vi "image_acquisitionBYModules.vi"() -> ()   [LabVIEW 2011]
uses:
  state.ctl
panel:
  out "Start acquisition 2":bool
  out "Output \nparameters 2":T2={"Frame rate (ms)"=2000, "Worm strain"="N2", "Time t"=0, "State"=enum."Image acquisition", "Time elapsed"=0.0, "Max_num_runs"=100000, "#TTL"=0, "SD start reference"=100000, "ImSub Value"=0, "Time of last TTL"=0, "Number of Columns"=2, "Number of Rows"=2, "# AdjacentTTL"=0, "Start sleep detection"="", "Sleep Detection"=FALSE, "# Sleep detections"=0, "Time of first sleep detection"=0, "Time max # adjacent TTL"=0, "Image t-1"=[], "Image t"=[]} {"Number of Rows" items=["1"=1, "2"=2, "3"=3, "4"=4]; "Number of Columns" items=["1"=1, "2"=2, "3"=3, "4"=4]}
  in  "Input\nparameters":T3={"Frame rate (ms)"=2000, "Worm Strain"="N2", "Time t"=0, "State"=enum."Image acquisition", "Acquisition time"=0.0, "Maximum # of images"=100000, "#TTL"=0, "time of third ttl "=100000, "ImSub Value"=0, "Time of last TTL"=0, "# Rows"=2, "# Columns"=2, "number of adjacentTTL"=0, "Sleep Deprivation status"="", "Sleep Detection"=FALSE, "Time of first sleep detection"=0, "# Sleep detections"=0, "Time max # adjacent TTL"=-10000, "Image t-1"=[], "Image t"=[]} {"# Columns" items=["1"=1, "2"=2, "3"=3, "4"=4]; "# Rows" items=["1"=1, "2"=2, "3"=3, "4"=4]}
  in  "Frame\nrate (ms)":u32=2000
  out "Intensity Graph 3":u16[][](graph)
  in  "Display\nImage 2":bool
  # "General settings"
  # "Select number of animals"
  # "Row"
  # "Column"
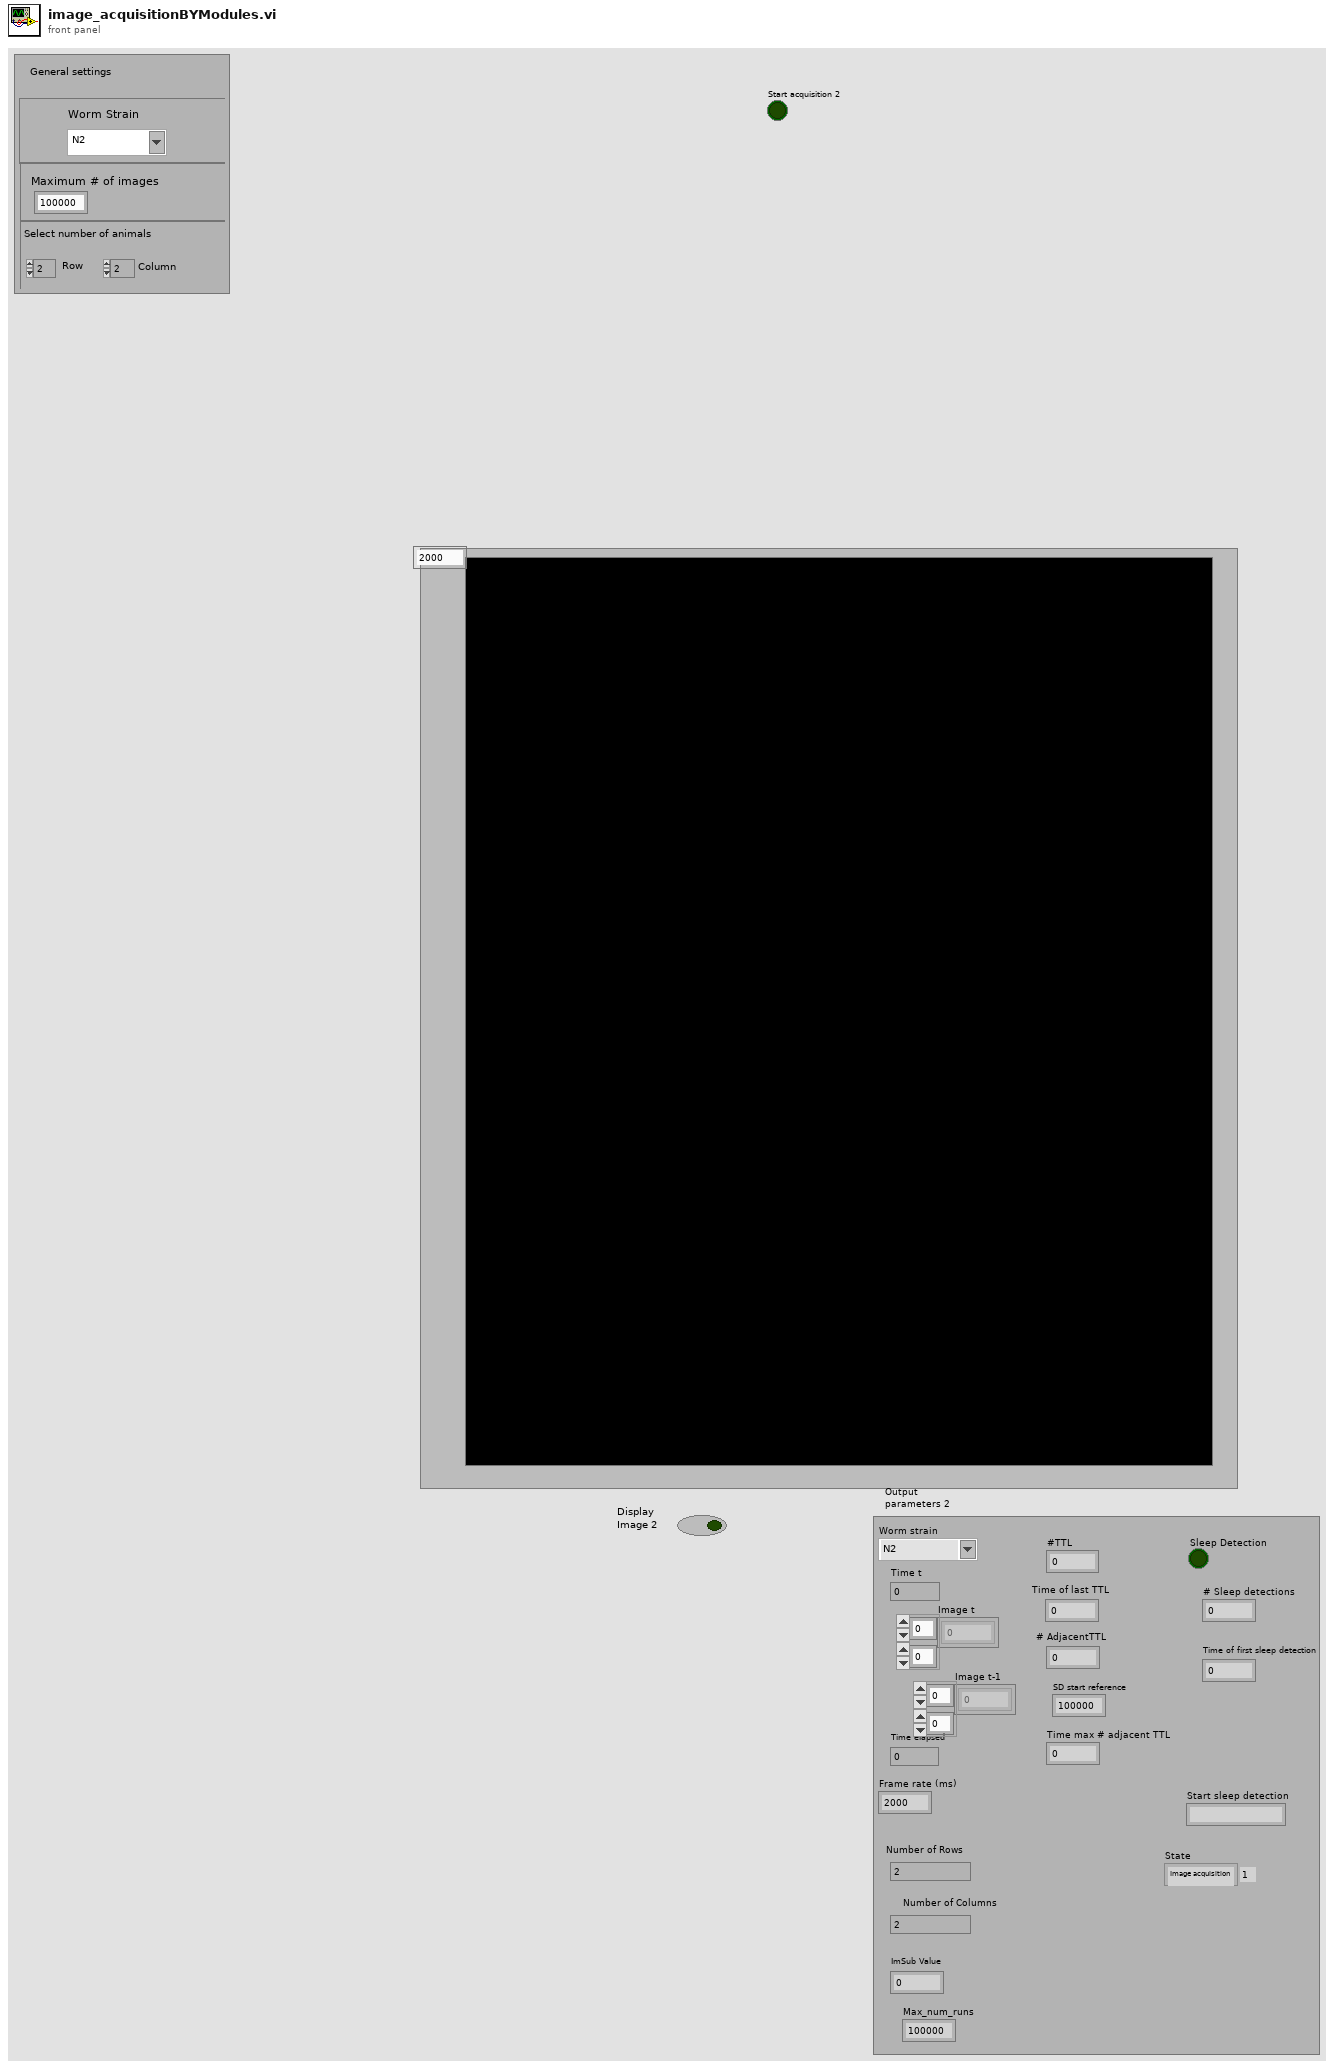
[diagram p1: front panel]
types:
  T1 = typedef "state.ctl" = enum16{"Initialize measurement", "Image acquisition", "Get image", "Save data", "Sleep detection", "Control TTL protocol ", "Sleep deprivation", "Update image", "Wait "}
  T2 = cluster{"Frame rate (ms)":u32, "Worm strain":string, "Time t":i32, "State":T1, "Time elapsed":dbl, "Max_num_runs":i32, "#TTL":i32, "SD start reference":i32, "ImSub Value":i32, "Time of last TTL":i32, "Number of Columns":u32, "Number of Rows":u32, "# AdjacentTTL":i32, "Start sleep detection":string, "Sleep Detection":bool, "# Sleep detections":i32, "Time of first sleep detection":i32, "Time max # adjacent TTL":i32, "Image t-1":i32[][], "Image t":i32[][]}
  T3 = cluster{"Frame rate (ms)":u32, "Worm Strain":string, "Time t":i32, "State":T1, "Acquisition time":dbl, "Maximum # of images":i32, "#TTL":i32, "time of third ttl ":i32, "ImSub Value":i32, "Time of last TTL":i32, "# Rows":u32, "# Columns":u32, "number of adjacentTTL":i32, "Sleep Deprivation status":string, "Sleep Detection":bool, "Time of first sleep detection":i32, "# Sleep detections":i32, "Time max # adjacent TTL":i32, "Image t-1":i32[][], "Image t":i32[][]}
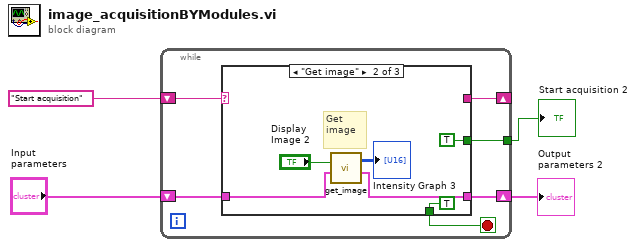
[diagram p0: block diagram]
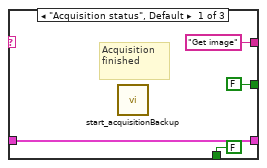
[diagram p2: hidden frame]
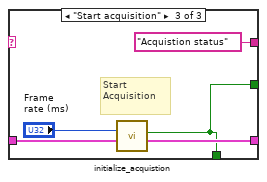
[diagram p3: hidden frame]
diagram:
  n1 = while {
    shift-right: [w9] -> _
    shift-left: "Start acquisition" -> [w10]
    shift-right: [w7] -> w2
    shift-left: "Input\nparameters" -> [w8]
    tunnel: [w5] -> w1
    stop <- w6 stop-if-true
    n2 = case shown="\"Get image\"" w10 {
      tunnel: ["Get image" _ "Acquistion status"] -> w9
      tunnel: w8 -> [w13 w18 w23]
      tunnel: [w13 w17 w22] -> w7
      tunnel: [FALSE ("Start acquisition") TRUE ("Start acquisition") w21] -> w6
      tunnel: [FALSE ("Start acquisition") TRUE ("Start acquisition") w21] -> w5
      frame "Acquisition status", Default {
        # "Acquisition\nfinished"
        n3 = call "start_acquisitionBackup.vi"() -> ()  [unwired: 12 in]
      }
      frame "Get image" {
        # "Get\nimage"
        n4 = call "get_image.vi"("Input\nparameters"=w18, 10:"Display\nImage 2") -> ("Output\nparameters"=w17:T3, "Intensity Graph"=→"Intensity Graph 3":u16[][])  [unwired: 8 in]
      }
      frame "Start acquisition" {
        # "Start\nAcquisition"
        n5 = call "initialize_acquistion.vi"("Input\nparameters"=w23, "Frame rate (ms)"="Frame\nrate (ms)") -> ("Output\nparameters"=w22:T3, "Start acquisition"=w21:bool)  [unwired: 8 in]
      }
    }
  }
  "Output \nparameters 2" <- w2
  "Start acquisition 2" <- w1
